vi "Time lapse wait for next frame - subvi.vi"() -> ()   [LabVIEW 2014]
uses:
  Shutter Control/Shutter SubVis/control shutters.ctl
  Shutter Control/Shutter SubVis/Global Shutter Variables - SubVI.vi
panel:
  in  "stop":bool
  in  "GO NOW!":bool
  in  "Pause":bool
  out "Time of this frame out (ms)":i32
  out "Sec. till next frame":ext(slide)
  out "Stopped?":bool
  in  "Time of last frame in":u32
  in  "Frame Interval (s)":dbl format="%#_13g"
  in  "Error In":errorcluster
  out "Error Out":errorcluster
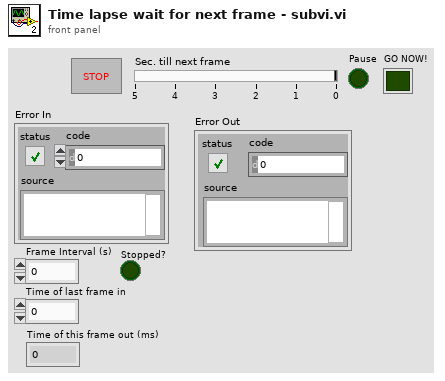
[diagram p1: front panel]
types:
  T1 = typedef "control shutters.ctl" = cluster{"Camera Shutter":bool, "Wheel Speed":u8, "Laser Shutter":enum32{"No Selection", "GFP", "Cy3 Long \nPass", "Cy3", "Cy5", "Off"}}
  T2 = enum32{"No Selection", "GFP", "Cy3 Long \nPass", "Cy3", "Cy5", "Off", "IR"}
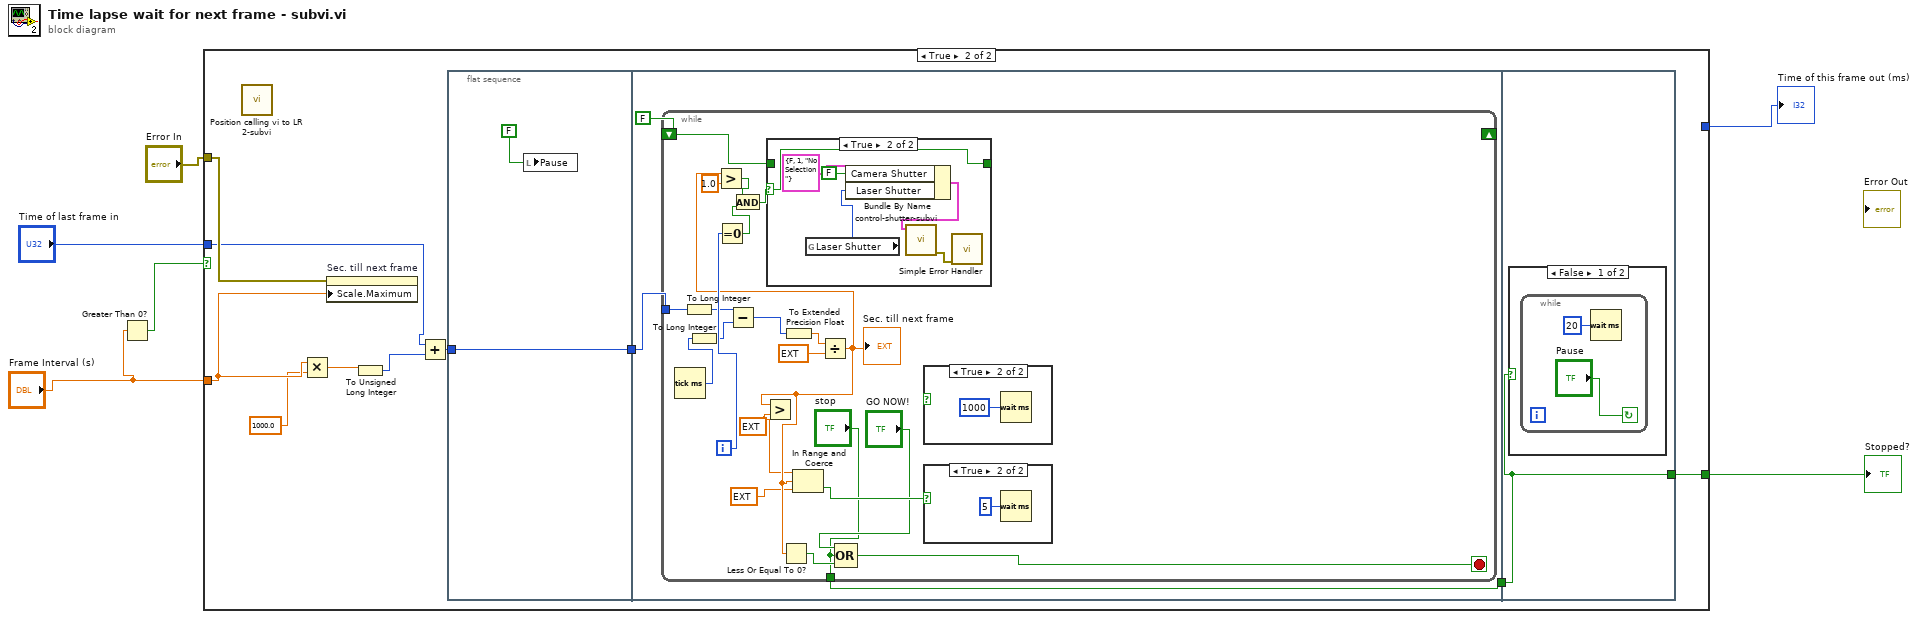
[diagram p0: block diagram]
diagram:
  n1 = Greater Than 0?(x="Frame Interval (s)") -> (x > 0?=w3:bool)
  n2 = case shown="True" w3 {
    tunnel: "Error In" -> [_ w17]
    tunnel: "Time of last frame in" -> [w7 w12]
    tunnel: "Frame Interval (s)" -> [_ w16]
    tunnel: [w7 _] -> w2
    tunnel: [_ w8] -> w1
    frame False {
    }
    frame True {
      n3 = call "Position calling vi to LR 2-subvi.vi"() -> ()  [unwired: 4 in, 2 out]
      n4 = Multiply(x=w16, y=1000.0) -> (x*y=w14:dbl)
      n5 = property on="Sec. till next frame" class="Slide (strict)"(error in=w17, "Scale.Maximum"=w16) -> ()  [unwired: 1 in, 2 out]
      n6 = To Unsigned Long Integer(number=w14) -> (unsigned 32bit integer=w13:u32)
      n7 = Add(x=w12, y=w13) -> (x+y=w10:u32)
      n8 = flat-sequence {
        tunnel: [w18] -> w11
        tunnel: w10 -> [w18]
        tunnel: w11 -> [w21]
        tunnel: [w20] -> w9
        tunnel: w9 -> [w53]
        tunnel: [w53] -> w8
        frame #0 {
          n9 = local write "Pause"(FALSE) -> ()
        }
        frame #1 {
          n10 = while {
            shift-right: _ -> [_]
            shift-left: FALSE -> [w43]
            tunnel: w21 -> [w33]
            tunnel: ["stop"] -> w20
            i -> [w39]
            stop <- w25 stop-if-true
            w29 = ext 1.04999999999999999996 ("y")
            n11 = Tick Count (ms)() -> (millisecond timer value=w37:u32)
            n12 = To Long Integer(number=w33) -> (32bit integer=w36:i32)
            n13 = To Long Integer(number=w37) -> (32bit integer=w35:i32)
            n14 = Equal To 0?(x=w39) -> (x = 0?=w40:bool)
            n15 = Subtract(x=w36, y=w35) -> (x-y=w34:i32)
            n16 = To Extended Precision Float(1:w34) -> (0:w32:ext)
            n17 = Divide(x=w32, y=ext 1000.0) -> (x/y=w30:ext)
            "Sec. till next frame" <- w30
            n18 = Greater?(x=w30, y=1.0) -> (0:w41:bool)
            n19 = And(x=w41, y=w40) -> (x .and. y?=w42:bool)
            n20 = Greater?(x=w30, y=w29) -> ()  [unwired: 1 out]
            n21 = case shown="True" w42 {
              selector: w42 -> [_ w47]
              tunnel: w43 -> [w46 _]
              tunnel: [w46 w47] -> _
              frame False {
              }
              frame True {
                n22 = global read "Global Shutter Variables - SubVI.vi" "Laser Shutter"() -> (w49:T2)
                n23 = Bundle By Name(cluster=T1 {"Camera Shutter"=FALSE, "Wheel Speed"=1, "Laser Shutter"=enum."No Selection"} ("Shutter Control"), "Camera Shutter"=FALSE, "Laser Shutter"=w49) -> (w51:T1)
                n24 = call "control-shutter-subvi.vi"("Shutter Control"=w51) -> ("Error Out"=w50:errorcluster)  [unwired: 10 in]
                n25 = call <vilib>:"Simple Error Handler.vi"("error in (no error)"=w50) -> ()  [unwired: 4 in, 5 out]
              }
            }
            n26 = Less Or Equal To 0?(x=w30) -> (x <= 0?=w26:bool)
            n27 = In Range and Coerce(upper limit=w29, x=w30, lower limit=ext 0.01 ("x/y")) -> (In Range?=w27:bool)  [unwired: 1 out]
            n28 = Compound Arithmetic op=OR("GO NOW!", "stop", w26) -> (w25:bool)
            n29 = case shown="True" {
              selector: _ -> [_ _]
              frame False {
              }
              frame True {
                n30 = Wait (ms)(milliseconds to wait=u32 1000) -> ()  [unwired: 1 out]
              }
            }
            n31 = case shown="True" w27 {
              frame False {
              }
              frame True {
                n32 = Wait (ms)(milliseconds to wait=u32 5) -> ()  [unwired: 1 out]
              }
            }
          }
        }
        frame #2 {
          n33 = case shown="False" w53 {
            frame False {
              n34 = while {
                stop <- "Pause" continue-if-true
                n35 = Wait (ms)(milliseconds to wait=u32 20) -> ()  [unwired: 1 out]
              }
            }
            frame True {
            }
          }
        }
      }
    }
  }
  "Stopped?" <- w1
  "Time of this frame out (ms)" <- w2
